vi "preform rotate op-poly.vi"   [LabVIEW 2019]
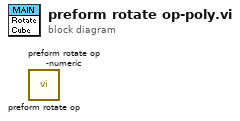
[diagram p0: block diagram]
diagram:
  n1 = call "preform rotate op.vi"() -> ()  [unwired: 9 in, 3 out]
  n2 = call "preform rotate op -numeric.vi"() -> ()  [unwired: 9 in, 3 out]
